vi "Array - Failure Message.vi"() -> ()   [LabVIEW 2017, in "Assertions.Tests.lvlib" / "Assert Collection Not Empty.lvlib"]
uses:
  Assert Collection Not Empty.lvlib
  7629c793-a7ff-4a62-891d-0070b4a98f08.vi
  src/Transparent Assertions/Constraints/Collection Is Empty/Collection Is Empty.lvclass
  C:/Users/pasca/Projects/Home/TransparentAssertions/src/Transparent Assertions/Constraints/Constraint/Constraint.lvclass
  src/Transparent Assertions/Constraints/LogicalNot/LogicalNot.lvclass
  src/Transparent Assertions/Constraints/UnaryOperator/UnaryOperator.lvclass
  src/Transparent Assertions/Assertions/Assertions.lvlib
panel:
  out "error out":errorcluster
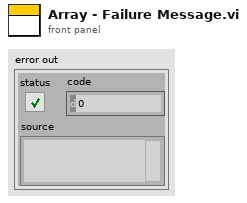
[diagram p1: front panel]
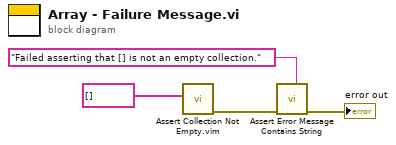
[diagram p0: block diagram]
diagram:
  n1 = call "Assert Collection Not Empty.vim"("Collection"=string[] []) -> ("error out"=w2:errorcluster)  [unwired: 10 in]
  n2 = call "Assert Error Message Contains String.vi"("Expected"="Failed asserting that [] is not an empty collection.", "error in (no error)"=w2) -> ("error out"=→"error out":errorcluster)  [unwired: 9 in]
